vi "Data Logging.vi"() -> ()   [LabVIEW 2016]
uses:
  <vilib>/Platform/TimedLoop/XDataNode/timing_clust.ctl
  <vilib>/Platform/TimedLoop/XDataNode/nitl_modes.ctl
  <vilib>/Platform/TimedLoop/XDataNode/wakeup.ctl
  Globale Variable/Globale Variable.vi
  <vilib>/Platform/TimedLoop/XDataNode/XDataNode.xnode
  <vilib>/Platform/TimedLoop/XDataNode/XDNodeRunTimeDep.lvlib
panel:
  in  "milliseconds to wait":u32=1
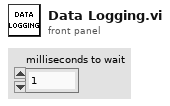
[diagram p1: front panel]
types:
  T1 = enum16{"open", "replace", "create", "open or create", "replace or create", "replace or create with confirmation"}
  T2 = typedef "XDNodeRunTimeDep.lvlib/timing_clust.ctl" = cluster{"Expected End [f-1]":u64, "Actual End [f-1]":u64, "Finished Late? [f-1]":bool, "Expected End [i-1]":u64, "Actual End [i-1]":u64, "Finished Late? [i-1]":bool, "Expected Start [i]":u64, "Actual Start [i]":u64, "Expected Start [f]":u64, "Actual Start [f]":u64, "Source Name":string, "Structure Name":string, "Period":i64, "Deadline":i64, "Offset":i64, "Start":i64, "Priority":i32, "Timeout":i32, "Mode":T3, "Wakeup Reason":T4, "Error":errorcluster, "Source Type":string, "Secondary Source Type":string, "Global End Time":u64, "Global Start Time":u64, "Frame Duration":u64, "Iteration Duration":u64, "Assigned CPU":i32, "I/O Scan Engine Mode":u32}
  T3 = typedef "XDNodeRunTimeDep.lvlib/nitl_modes.ctl" = enum32{"No Change", "Process missed periods, maintain original phase", "Discard missed periods, maintain original phase", "Process missed periods, ignore original phase", "Discard missed periods, ignore original phase"}
  T4 = typedef "XDNodeRunTimeDep.lvlib/wakeup.ctl" = enum32{"Normal", "Aborted", "Asynchronous wakeup", "Timing source error", "Timed loop error", "Timeout"}
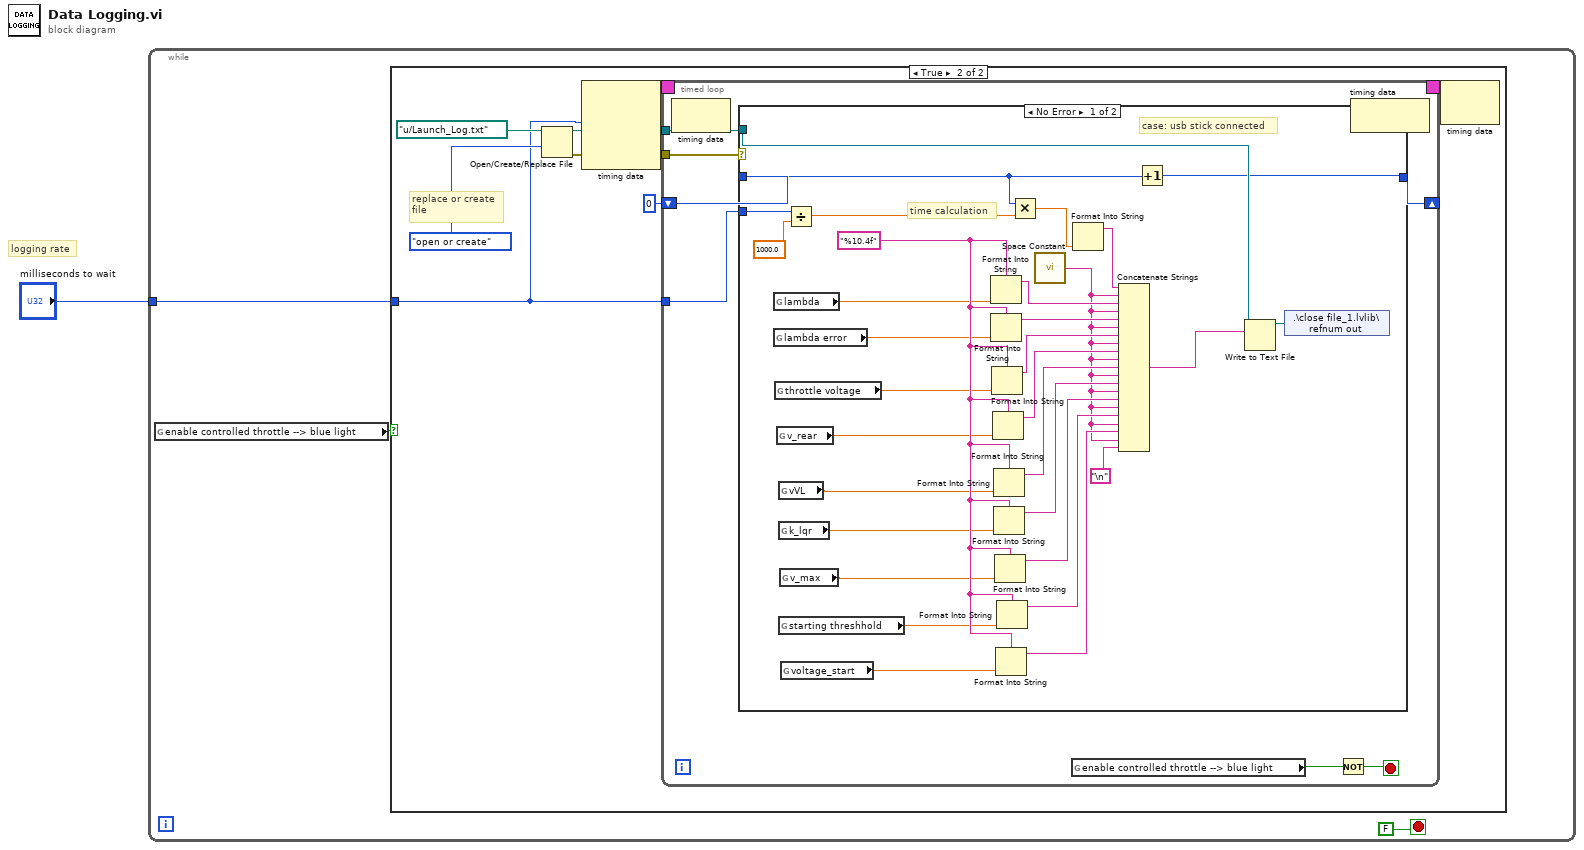
[diagram p0: block diagram]
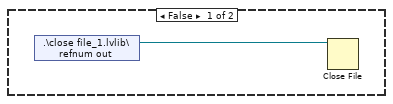
[diagram p2: hidden frame]
diagram:
  # "logging rate"
  n1 = while {
    tunnel: "milliseconds to wait" -> [w4]
    stop <- FALSE stop-if-true
    n2 = global read "Globale Variable.vi" "enable controlled throttle --> blue light"() -> (w3:bool)
    n3 = case shown="True" w3 {
      tunnel: w4 -> [_ w6]
      frame False {
        n4 = shared-variable ".\\close file_1.lvlib\\refnum out"() -> (w5:refnum<file>)  [unwired: 1 in, 1 out]
        n5 = Close File(refnum=w5) -> ()  [unwired: 1 in, 2 out]
      }
      frame True {
        # "replace or create \nfile"
        n6 = Open/Create/Replace File(file path (use dialog)=path "u:/Launch_Log.txt", operation (0:open)=T1."open or create") -> (refnum out=w11:refnum<file>, error out=w9:errorcluster)  [unwired: 4 in, 1 out]
        n7 = node-c288(w6) -> (w8:T2)  [unwired: 3 in]
        n8 = timed-loop {
          tunnel: w11 -> [w20]
          shift-right: [w18] -> _
          shift-left: 0 -> [w19]
          tunnel: w9 -> [w17]
          tunnel: w6 -> [w16]
          timing: w8 -> [_]
          timing-out: [_] -> w7
          stop <- w15 stop-if-true
          n9 = node-c288() -> ()  [unwired: 1 in, 1 out]
          n10 = case shown="No Error" w17 {
            tunnel: w20 -> [w52 _]
            tunnel: w19 -> [w25 w54]
            tunnel: [w51 w54] -> w18
            tunnel: w16 -> [w27 _]
            frame No Error {
              w41 = "%10.4f" ("format string")
              # "time calculation"
              # "case: usb stick connected"
              n11 = global read "Globale Variable.vi" "lambda"() -> (w37:dbl)
              n12 = global read "Globale Variable.vi" "lambda error"() -> (w36:dbl)
              n13 = global read "Globale Variable.vi" "throttle voltage"() -> (w35:dbl)
              n14 = global read "Globale Variable.vi" "v_rear"() -> (w34:dbl)
              n15 = global read "Globale Variable.vi" "vVL"() -> (w33:dbl)
              n16 = global read "Globale Variable.vi" "k_lqr"() -> (w32:dbl)
              n17 = global read "Globale Variable.vi" "starting threshhold"() -> (w30:dbl)
              n18 = global read "Globale Variable.vi" "v_max"() -> (w31:dbl)
              n19 = global read "Globale Variable.vi" "voltage_start"() -> (w29:dbl)
              n20 = Divide(x=w27, y=1000.0) -> (x/y=w26:dbl)
              n21 = Format Into String(format string=w41, w37) -> (resulting string=w45:string)  [unwired: 2 in, 1 out]
              n22 = Format Into String(format string=w41, w36) -> (resulting string=w46:string)  [unwired: 2 in, 1 out]
              n23 = Format Into String(format string=w41, w35) -> (resulting string=w47:string)  [unwired: 2 in, 1 out]
              n24 = Format Into String(format string=w41, w34) -> (resulting string=w48:string)  [unwired: 2 in, 1 out]
              n25 = Format Into String(format string=w41, w33) -> (resulting string=w49:string)  [unwired: 2 in, 1 out]
              n26 = Format Into String(format string=w41, w32) -> (resulting string=w44:string)  [unwired: 2 in, 1 out]
              n27 = Format Into String(format string=w41, w31) -> (resulting string=w43:string)  [unwired: 2 in, 1 out]
              n28 = Format Into String(format string=w41, w29) -> (resulting string=w40:string)  [unwired: 2 in, 1 out]
              n29 = Format Into String(format string=w41, w30) -> (resulting string=w42:string)  [unwired: 2 in, 1 out]
              n30 = Multiply(x=w25, y=w26) -> (x*y=w24:dbl)
              n31 = call <vilib>:"Space Constant.vi"() -> ("String"=w39:string)
              n32 = Format Into String(w24) -> (resulting string=w50:string)  [unwired: 3 in, 1 out]
              n33 = Concatenate Strings(w50, w39, w45, w39, w46, w39, w47, w39, w48, w39, w49, w39, w44, w39, w43, w39, w42, w39, w40, w39, "\n") -> (w53:string)
              n34 = Increment(x=w25) -> (x+1=w51:i32)
              n35 = Write to Text File(file (use dialog)=w52, text=w53) -> (refnum out=w23:refnum<file>)  [unwired: 2 in, 2 out]
              n36 = shared-variable ".\\close file_1.lvlib\\refnum out"(w23) -> ()  [unwired: 1 in, 1 out]
            }
            frame Error {
            }
          }
          n37 = global read "Globale Variable.vi" "enable controlled throttle --> blue light"() -> (w14:bool)
          n38 = Not(x=w14) -> (.not. x?=w15:bool)
          n39 = node-c288() -> ()  [unwired: 1 in, 1 out]
        }
        n40 = node-c288(w7) -> ()  [unwired: 1 out]
      }
    }
  }
